vi "Stop Core.vi"(10 "final error code":i32, 11 "CS++BaseActor in":refnum<class "CS++BaseActor.lvclass">) -> (3 "CS++BaseActor out":refnum<class "CS++BaseActor.lvclass">)   [LabVIEW 2013, in "CS++BaseActor.lvlib" / "CS++BaseActor.lvclass"]
doc: "(<B>Filename</B>: Actor Framework.lvlib:Actor.lvclass:Stop Core.vi)\n\nDefines what the actor does before it stops. Use the <B>final error code</B> input to determine whether the actor shut down in response to an error.\n\nBy default, this method does nothing. A descendant class may override it to define behavior, such as shutting down any processes the actor initiated in its override of the Actor Core method."
uses:
  CS++BaseActor.lvclass
  <userlib>/Monitored Actor/Actor/Monitored Actor.lvclass
  CS++BaseActor.lvclass/CS++BaseActor.ctl
  <vilib>/ActorFramework/Message Enqueuer/Message Enqueuer.lvclass/Message Enqueuer.ctl
  <vilib>/ActorFramework/Message Enqueuer/Enqueue.vi
  <vilib>/ActorFramework/Message Priority Queue/Priority Enqueue.vi
  <vilib>/ActorFramework/Stop Msg/Stop Msg.lvclass
  Libraries/MessageLogger/CS++MessageLogger.lvlib
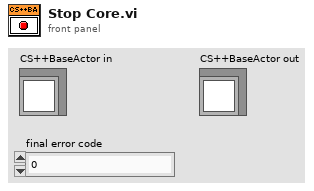
[diagram p1: front panel]
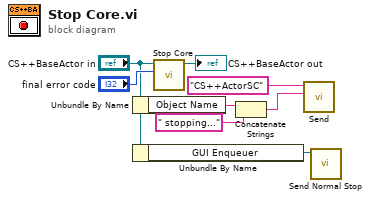
[diagram p0: block diagram]
diagram:
  n1 = Unbundle By Name("CS++BaseActor in") -> ("Object Name"=w4:string)
  n2 = Unbundle By Name("CS++BaseActor in") -> ("GUI Enqueuer"=w2:refnum<class "Message Enqueuer.lvclass">)
  n3 = call-parent "Stop Core.vi"("final error code"="final error code", "Monitored Actor in"="CS++BaseActor in") -> ("Monitored Actor out"=→"CS++BaseActor out":refnum<class "CS++BaseActor.lvclass">)  [unwired: 9 in]
  n4 = Concatenate Strings(w4, " stopping..." ("string")) -> (w5:string)
  n5 = call "Send.vi"("Message Content"=w5, "Message Tag"="CS++ActorSC") -> ()  [unwired: 9 in, 1 out]
  n6 = call <vilib>:"Send Normal Stop.vi"("Message Enqueuer"=w2) -> ()  [unwired: 10 in, 1 out]
